vi "GT_StepDir.vi"(2 "Step in":i16, 3 "rtn_In":cluster{"rtn":i16, "Func":string}) -> (0 "Step out":i16, 1 "rtn_Out":cluster{"rtn":i16, "Func":string})   [LabVIEW 2014]
uses:
  VC6/gts.dll
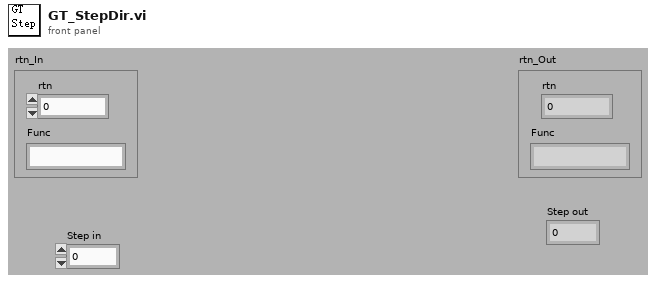
[diagram p1: front panel]
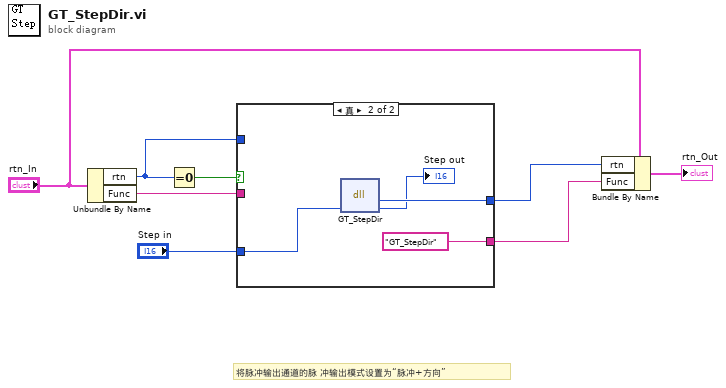
[diagram p0: block diagram]
diagram:
  # "将脉冲输出通道的脉 冲输出模式设置为“脉冲+方向”"
  n1 = Unbundle By Name("rtn_In") -> ("rtn"=w2:i16, "Func"=w1:string)
  n2 = Equal To 0?(x=w2) -> (x = 0?=w8:bool)
  n3 = case shown="真" w8 {
    tunnel: "Step in" -> [_ w14]
    tunnel: [w10 w13] -> w5
    tunnel: [w9 "GT_StepDir" ("Func")] -> w4
    tunnel: w2 -> [w10 _]
    tunnel: w1 -> [w9 _]
    frame False {
    }
    frame True {
      n4 = dll-call lib="PTH2Fabs DNewGTS AC-800LWin7版源程序-20170926gts85VC6gts.dll" fn="GT_StepDir"("Step"=w14) -> ("rtn"=w13:i16, "Step"=→"Step out":i16)  [unwired: 3 in, 2 out]
    }
  }
  n5 = Bundle By Name(cluster="rtn_In", "rtn"=w5, "Func"=w4) -> (→"rtn_Out":cluster{"rtn":i16, "Func":string})
